vi "Do.vi"(8 "error in (no error)":errorcluster, 10 "Actor in":refnum<class "Actor.lvclass">, 11 "TreeList Task Msg":refnum<class "TreeList Task Msg.lvclass">) -> (0 "error out":errorcluster, 2 "Actor out":refnum<class "Actor.lvclass">)   [LabVIEW 2016, in "TreeList Actor.lvlib" / "TreeList Task Msg.lvclass"]
uses:
  TreeList Task Msg.lvclass
  <vilib>/ActorFramework/Actor/Actor.lvclass
  TreeList/TreeList.lvclass
  E:/Program Files (x86)/National Instruments/LabVIEW 2016/vi.lib/ActorFramework/Actor/Actor.lvclass
  TreeList Task Msg.lvclass/TreeList Task Msg.ctl
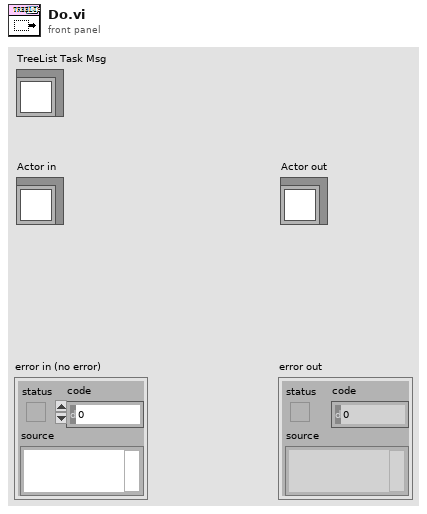
[diagram p1: front panel]
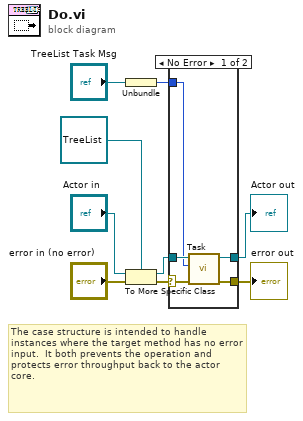
[diagram p0: block diagram]
diagram:
  # "The case structure is intended to handle instances where the target method has no error input.  It both prevents the operation and protects error throughput back to the actor core."
  n1 = Unbundle("TreeList Task Msg") -> (w1:i32)
  n2 = To More Specific Class(target class=refnum<class "TreeList.lvclass"> refnum ("Actor in"), reference="Actor in", error in="error in (no error)") -> (specific class reference=w8:refnum<class "TreeList.lvclass">, error out=w4:errorcluster)
  n3 = case shown="No Error" w4 {
    selector: w4 -> [w11 w16]
    tunnel: w8 -> [w14 w15]
    tunnel: [w13 w16] -> w3
    tunnel: [w12 w15] -> w2
    tunnel: w1 -> [w10 _]
    frame No Error {
      n4 = call-dynamic "Task.vi"("error in (no error)"=w11, "Data"=w10, "TreeList in"=w14) -> ("error out"=w13:errorcluster, "TreeList out"=w12:refnum<class "TreeList.lvclass">)  [unwired: 7 in]
    }
    frame Error {
    }
  }
  "error out" <- w3
  "Actor out" <- w2
